vi "CreatePluginTreeShortcutMenu.vi"(8 "error in (no error)":errorcluster, 10 "Tag":string, 11 "Menu in":refnum<k9>) -> (0 "error out":errorcluster)   [LabVIEW 2018]
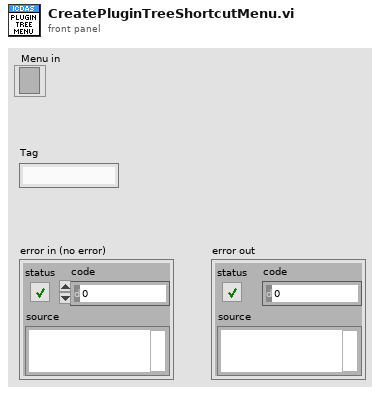
[diagram p1: front panel]
types:
  T1 = typedef "Plugin Tree Tag.ctl" = cluster{"ItemType":T2, "Name":string, "Path":path, "Script":string[]}
  T2 = typedef "Plugins Tree Item Type.ctl" = enum16{"Plugin", "Instrument", "INI File", "INI Script"}
  T3 = typedef "cntlRefs.ctl" = cluster{"rngFGen":refnum<vi>, "rngDigitizer":refnum<vi>, "btnHide":refnum<vi>, "rngInst":refnum<vi>, "Instrument Modules":refnum<vi>, "RelativePathToINIFiles ":refnum<vi>, "PluginTree":refnum<vi>, "TestListboxRef":refnum<vi>, "path.tstFile":refnum<vi>, "cmbxRunningModules":refnum<vi>, "TestDataSubPanel":refnum<vi>, "TestDataCaption":refnum<vi>, "btnPopInOut":refnum<vi>, "PluginMgrQ":refnum<queue>, "TestMgrQ":refnum<queue>, "TestMgrSubPanel":refnum<vi>, "PluginMgrSubPanel":refnum<vi>, "PwrReqHandle":u32, "btnStopOneTest":refnum<vi>, "pathUserfiles":refnum<vi>, "PluginTreeCaption":refnum<vi>, "MainVIRef":refnum<vi>, "btnStatus":refnum<vi>}
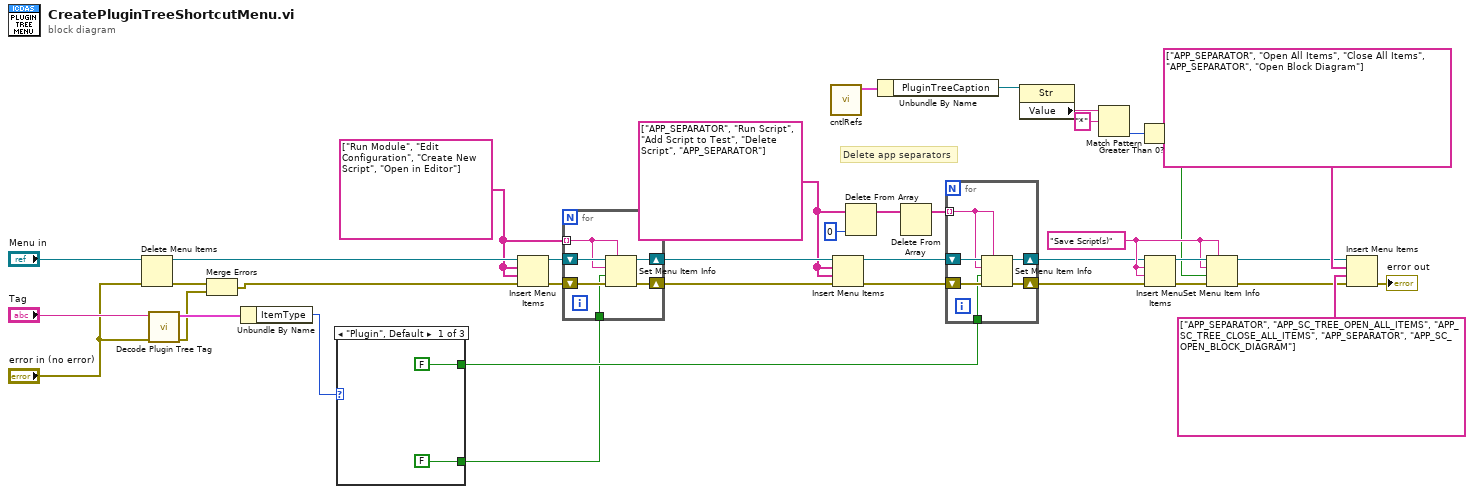
[diagram p0: block diagram]
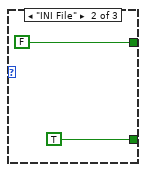
[diagram p2: hidden frame]
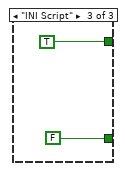
[diagram p3: hidden frame]
diagram:
  w7 = string[] ["Run Module", "Edit Configuration", "Create New Script", "Open in Editor"] ("regular expression")
  w4 = string[] ["APP_SEPARATOR", "Run Script", "Add Script to Test", "Delete Script", "APP_SEPARATOR"]
  w25 = "Save Script(s)"
  # "Delete app separators"
  n1 = Delete Menu Items(6:"error in (no error)", 9:"Menu in") -> (0:w34:errorcluster, 3:w11:refnum<k9>)  [unwired: 2 in]
  n2 = call "Decode Plugin Tree Tag.vi"("error in (no error)"="error in (no error)", "Tag"="Tag") -> ("error out"=w33:errorcluster, "Plugin Tree Tag"=w36:T1)  [unwired: 8 in]
  n3 = Merge Errors(w34, w33) -> (w32:errorcluster)
  n4 = Unbundle By Name(w36) -> ("ItemType"=w18:T2)
  n5 = case shown="\"Plugin\", Default" w18 {
    tunnel: [FALSE TRUE FALSE] -> w6
    tunnel: [FALSE FALSE TRUE] -> w13
    frame "Plugin", Default {
    }
    frame "INI File" {
    }
    frame "INI Script" {
    }
  }
  n6 = Insert Menu Items(6:w32, 7:w7, 8:w7, 9:w11) -> (0:w12:errorcluster, 3:w9:refnum<k9>)  [unwired: 2 in, 1 out]
  n7 = for {
    shift-right: [w49] -> w10
    shift-left: w12 -> [w50]
    shift-right: [w47] -> w8
    shift-left: w9 -> [w48]
    tunnel: w7 -> [w46] mode=indexing
    tunnel: w6 -> [w45]
    n8 = Set Menu Item Info(7:w46, 8:w50, 9:w45, 10:w46, 11:w48) -> (0:w49:errorcluster, 3:w47:refnum<k9>)  [unwired: 2 in]
  }
  n9 = call "cntlRefs.vi"() -> ("cntlRefs"=w24:T3)  [unwired: 10 in, 1 out]
  n10 = Insert Menu Items(6:w10, 7:w4, 8:w4, 9:w8) -> (0:w17:errorcluster, 3:w15:refnum<k9>)  [unwired: 2 in, 1 out]
  n11 = Delete From Array(array=w4, index=0) -> (array with subset deleted=w1:string[])  [unwired: 1 in, 1 out]
  n12 = Unbundle By Name(w24) -> ("PluginTreeCaption"=w23:refnum<vi>)
  n13 = Delete From Array(array=w1) -> (array with subset deleted=w2:string[])  [unwired: 2 in, 1 out]
  n14 = for {
    shift-right: [w55] -> w16
    shift-left: w17 -> [w56]
    shift-right: [w53] -> w14
    shift-left: w15 -> [w54]
    tunnel: w2 -> [w52] mode=indexing
    tunnel: w13 -> [w51]
    n15 = Set Menu Item Info(7:w52, 8:w56, 9:w51, 10:w52, 11:w54) -> (0:w55:errorcluster, 3:w53:refnum<k9>)  [unwired: 2 in]
  }
  n16 = property class="Str"(reference=w23) -> ("Value"=w22:string)  [unwired: 1 in, 2 out]
  n17 = Match Pattern(string=w22, regular expression="*") -> (offset past match=w20:i32)  [unwired: 1 in, 3 out]
  n18 = Greater Than 0?(x=w20) -> (x > 0?=w19:bool)
  n19 = Insert Menu Items(6:w16, 7:w25, 8:w25, 9:w14) -> (0:w31:errorcluster, 3:w27:refnum<k9>)  [unwired: 2 in, 1 out]
  n20 = Set Menu Item Info(7:w25, 8:w31, 9:w19, 10:w25, 11:w27) -> (0:w28:errorcluster, 3:w26:refnum<k9>)  [unwired: 2 in]
  n21 = Insert Menu Items(6:w28, 7:string[] ["APP_SEPARATOR", "APP_SC_TREE_OPEN_ALL_ITEMS", "APP_SC_TREE_CLOSE_ALL_ITEMS", "APP_SEPARATOR", "APP_SC_OPEN_BLOCK_DIAGRAM"] ("submenu tags"), 8:string[] ["APP_SEPARATOR", "Open All Items", "Close All Items", "APP_SEPARATOR", "Open Block Diagram"] ("submenu tags"), 9:w26) -> (0:→"error out":errorcluster)  [unwired: 2 in, 2 out]
